vi "set dependency.vi"(8 "error in (no error)":errorcluster, 11 "Device Item Ref in":T1 format="%.0x") -> (0 "error out":errorcluster)   [LabVIEW 2017, in "Data Sharing Framework System Explorer.lvlib"]
uses:
  Data Sharing Framework System Explorer.lvlib
  <vilib>/NI Veristand/Custom Device API/Custom Device Item Ref.ctl
  <vilib>/NI Veristand/Custom Device API/Custom Device File Dependency.ctl
  <vilib>/NI Veristand/Custom Device API/Path Specification.ctl
  <vilib>/NI Veristand/Custom Device API/Path Type.ctl
  <vilib>/NI Veristand/Custom Device API/Custom Device Supported Target.ctl
  <vilib>/NI VeriStand/Custom Device API/Custom Device API.lvlib
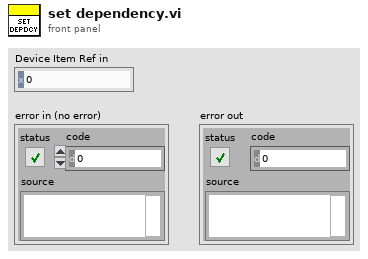
[diagram p1: front panel]
types:
  T1 = typedef "Custom Device API.lvlib/Custom Device Item Ref.ctl" = u64
  T2 = typedef "Custom Device API.lvlib/Custom Device Supported Target.ctl" = enum16{"All", "PharLap", "VxWorks", "Windows", "Linux_32_ARM", "Linux_x64", "PharLap & Windows", "PharLap & VxWorks", "VxWorks & Windows"}
  T3 = typedef "Custom Device API.lvlib/Path Type.ctl" = enum16{"Absolute", "To Base", "To Common Data Dir", "To Application Data Dir"}
  T4 = typedef "Custom Device API.lvlib/Custom Device File Dependency.ctl" = cluster{"Source":T5, "RT Destination":path, "ForceDownload?":bool, "SupportedTarget":T2, "Version":string}
  T5 = typedef "Custom Device API.lvlib/Path Specification.ctl" = cluster{"Path":path, "Type":T3}
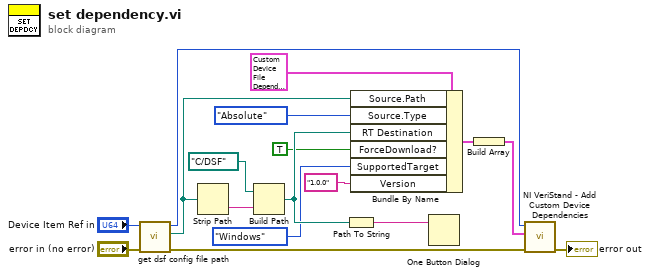
[diagram p0: block diagram]
diagram:
  n1 = call "get dsf config file path.vi"("error in (no error)"="error in (no error)", "Node Ptr"="Device Item Ref in") -> ("error out"=w17:errorcluster, "Path"=w9:path, "Item Ref out"=w12:T1)  [unwired: 7 in]
  n2 = Strip Path(path=w9) -> (name=w2:string)  [unwired: 1 out]
  n3 = Build Path(base path=path "C:/DSF" ("RT Destination"), name or relative path=w2) -> (appended path=w14:path)
  n4 = Path To String(path=w14) -> (string=w15:string)
  n5 = Bundle By Name(cluster=T4 {"Source"={"Path"=path "", "Type"=enum."Absolute"}, "RT Destination"=path "", "ForceDownload?"=FALSE, "SupportedTarget"=enum."PharLap", "Version"=""} ("element"), "Source.Path"=w9, "Source.Type"=Path_Type."Absolute", "RT Destination"=w14, "ForceDownload?"=TRUE, "SupportedTarget"=Custom_Device_Supported_Target."Windows", "Version"="1.0.0") -> (w7:T4)
  n6 = One Button Dialog(message=w15) -> ()  [unwired: 1 in, 1 out]
  n7 = Build Array(w7) -> (w8:T4[])
  n8 = call <vilib>:"NI VeriStand - Add Custom Device Dependencies.vi"("error in (no error)"=w17, "Dependencies"=w8, "Device Ref in"=w12) -> ("error out"=→"error out":errorcluster)  [unwired: 7 in, 1 out]
